vi "Get File Extension.vi"(8 "error in (no error)":errorcluster, 11 "file":path) -> (0 "error out":errorcluster, 1 "filename without extension":string, 2 "lowercase file extension":string, 3 "dup file":path)   [LabVIEW 2009]
doc: "Returns the file extension of a file you specify."
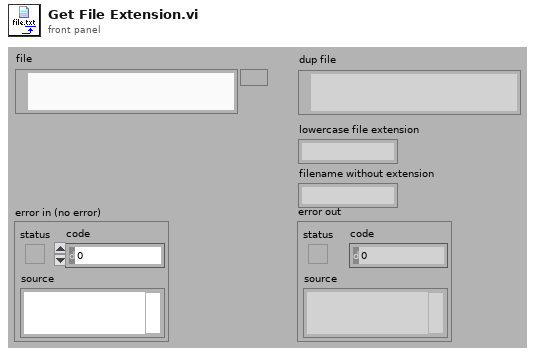
[diagram p1: front panel]
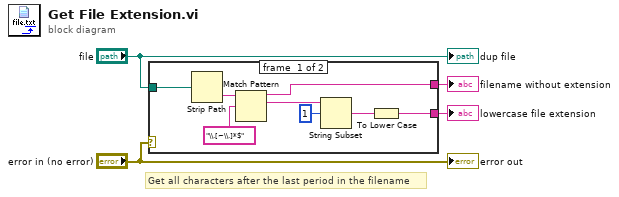
[diagram p0: block diagram]
diagram:
  # "Get all characters after the last period in the filename"
  n1 = case shown="No Error" "error in (no error)" {
    tunnel: "file" -> [w11 _]
    tunnel: [w9 _] -> w2
    tunnel: [w5 _] -> w1
    frame #0 {
      n2 = Strip Path(path=w11) -> (name=w10:string)  [unwired: 1 out]
      n3 = Match Pattern(string=w10, regular expression="\\.[~\\.]*$") -> (before substring=w5:string, match substring=w12:string)  [unwired: 3 out]
      n4 = String Subset(string=w12, offset (0)=1) -> (substring=w8:string)  [unwired: 1 out]
      n5 = To Lower Case(string=w8) -> (all lower case string=w9:string)
    }
    frame #1 {
    }
  }
  "lowercase file extension" <- w2
  "filename without extension" <- w1
  "error out" <- "error in (no error)"
  "dup file" <- "file"
